vi "_Lookup Channel.vi"(8 "error in (no error)":errorcluster, 10 "Channel Name":string, 11 "Loop Data 2":T1) -> (0 "error out":errorcluster, 1 "Index":i32, 2 "Group":refnum<class "Group.lvclass">, 3 "Loop Data 3":T1, 4 "Data Type":T2)   [LabVIEW 2020, in "Vecto.lvlib" / "ChannelService.lvclass"]
uses:
  ChannelService.lvclass
  Group/Group.lvclass
  Group Data Type.ctl
  Loop Data.ctl
  Group/Group.lvclass/Group.ctl
  Group Config/Group Config.lvclass/Group Config.ctl
  Group Config/Group Data Type.vi
  VectoConfig/VectoConfig.lvlib
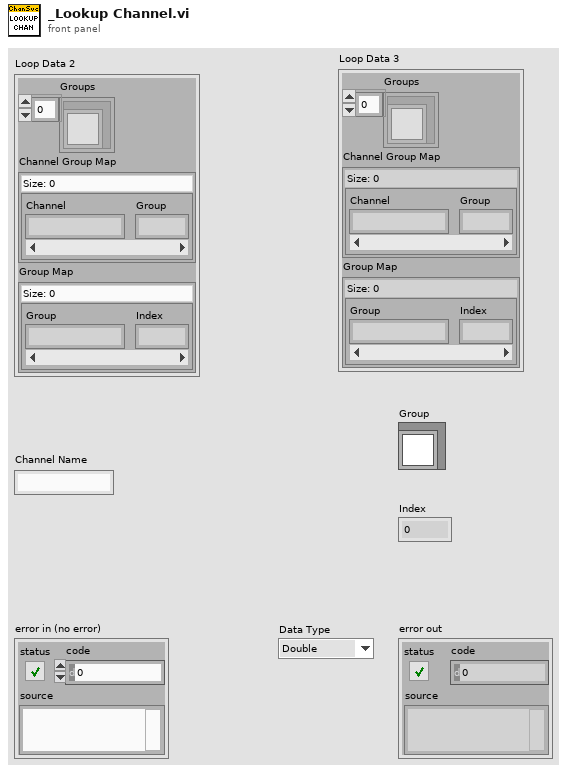
[diagram p1: front panel]
types:
  T1 = typedef "Vecto.lvlib/ChannelService.lvclass/Loop Data.ctl" = cluster{"Groups":refnum<class "Group.lvclass">[], "Channel Group Map":map{string, i32}, "Group Map":map{string, i32}}
  T2 = typedef "VectoConfig.lvlib/Group Data Type.ctl" = enum16{"Double", "String", "Bool"}
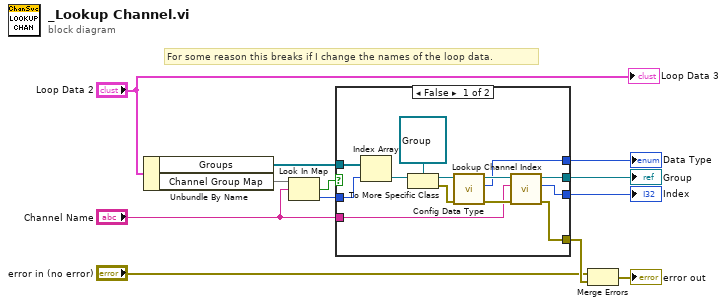
[diagram p0: block diagram]
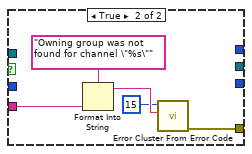
[diagram p2: hidden frame]
diagram:
  # "For some reason this breaks if I change the names of the loop data."
  n1 = Unbundle By Name("Loop Data 2") -> ("Groups"=w9:refnum<class "Group.lvclass">[], "Channel Group Map"=w12:map{string, i32})
  n2 = Look In Map(map=w12, key="Channel Name") -> (key not found?=w11:bool, value=w10:i32)  [unwired: 1 in]
  n3 = case shown="False" w11 {
    tunnel: w10 -> [w23 _]
    tunnel: w9 -> [w24 _]
    tunnel: "Channel Name" -> [w20 w30]
    tunnel: [w18 _] -> w7
    tunnel: [w19 w26] -> w6
    tunnel: [w17 _] -> w3
    tunnel: [w13 _] -> w2
    frame False {
      n4 = Index Array(array=w24, index=w23) -> (element=w22:refnum<class "Group.lvclass">)
      n5 = To More Specific Class(target class=refnum<class "Group.lvclass"> refnum ("Vecto.lvlib:GroupAbstract.lvclass"), reference=w22) -> (specific class reference=w16:refnum<class "Group.lvclass">, error out=w14:errorcluster)  [unwired: 1 in]
      n6 = call "Config Data Type.vi"("error in (no error)"=w14, "Group in"=w16) -> ("error out"=w25:errorcluster, "Group Data Type"=w13:T2, "Group out"=w15:refnum<class "Group.lvclass">)  [unwired: 7 in]
      n7 = call "Lookup Channel Index.vi"("error in (no error)"=w25, "Channel Name"=w20, "Group in"=w15) -> ("error out"=w19:errorcluster, "Index"=w17:i32, "Group out"=w18:refnum<class "Group.lvclass">)  [unwired: 6 in]
    }
    frame True {
      n8 = Format Into String(format string="Owning group was not found for channel \"%s\"", w30) -> (resulting string=w28:string)  [unwired: 2 in, 1 out]
      n9 = call <vilib>:"Error Cluster From Error Code.vi"("error message (\"\")"=w28, "error code (0)"=15) -> ("error out"=w26:errorcluster)  [unwired: 7 in]
    }
  }
  "Group" <- w7
  "Index" <- w3
  "Data Type" <- w2
  n10 = Merge Errors("error in (no error)", w6) -> (→"error out":errorcluster)
  "Loop Data 3" <- "Loop Data 2"
